vi "Format Group String.vi"(8 "error in":errorcluster, 10 "Modbus Type":T2, 11 "VS Type":T1) -> (0 "error out":errorcluster, 3 "Group String":string)   [LabVIEW 2020, in "Modbus Master System Explorer.lvlib"]
uses:
  System Explorer/Modbus Master System Explorer.lvlib
  System Explorer/SubVIs/Modbus Type.ctl
  <vilib>/NI VeriStand/Custom Device API/Custom Device Channel Type.ctl
  Modbus Master Shared.lvlib
  <vilib>/NI VeriStand/Custom Device API/Custom Device API.lvlib
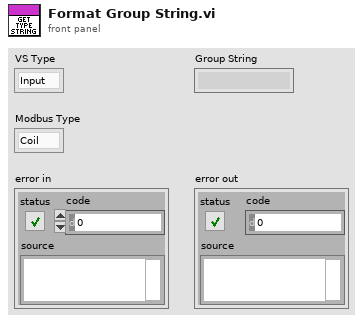
[diagram p1: front panel]
types:
  T1 = typedef "Custom Device API.lvlib/Custom Device Channel Type.ctl" = enum16{"Input", "Output"}
  T2 = typedef "Modbus Master Shared.lvlib/Modbus Type.ctl" = enum16{"Coil", "Discrete Input", "Holding Register", "Input Register"}
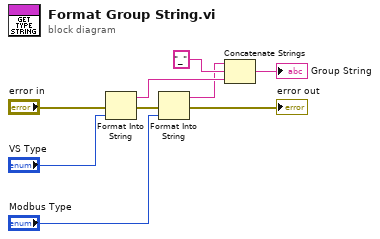
[diagram p0: block diagram]
diagram:
  n1 = Format Into String(error in="error in", "VS Type") -> (resulting string=w5:string, error out=w6:errorcluster)  [unwired: 2 in]
  n2 = Format Into String(error in=w6, "Modbus Type") -> (resulting string=w3:string, error out=→"error out":errorcluster)  [unwired: 2 in]
  n3 = Concatenate Strings(w3, "_", w5) -> (→"Group String":string)
